vi "Do Request.vi"(7 "Processing In":refnum<class "Processing.lvclass">, 11 "Test HTTPS Controller in":refnum<class "Test HTTPS Controller.lvclass">) -> (0 "error out":errorcluster, 5 "Processing":refnum<class "Processing.lvclass">)   [LabVIEW 2020, in "Test HTTPS Controller.lvclass"]
uses:
  Test HTTPS Controller.lvclass
  HTTP Server/Processing/Processing.lvclass
  HTTP Server/Processing/Processing.lvclass/Processing.ctl
  <vilib>/IlluminatedG/IG HTTP Utils/HTTP Utils/Response/Response.lvclass
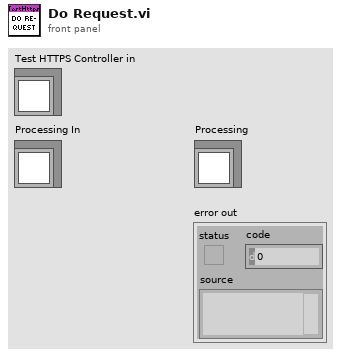
[diagram p1: front panel]
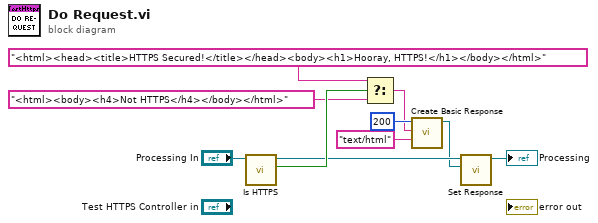
[diagram p0: block diagram]
diagram:
  n1 = call "Is HTTPS.vi"("Processing in"="Processing In") -> ("HTTPS?"=w9:bool, "Processing out"=w4:refnum<class "Processing.lvclass">)  [unwired: 8 in, 1 out]
  n2 = Select(t="<html><head><title>HTTPS Secured!</title></head><body><h1>Hooray, HTTPS!</h1></body></html>", s=w9, f="<html><body><h4>Not HTTPS</h4></body></html>") -> (s? t:f=w5:string)
  n3 = call <vilib>:"Create Basic Response.vi"("Content-Type (text/plain)"="text/html", "Payload"=w5, "Status Code"=u16 200) -> ("Response out"=w3:refnum<class "Response.lvclass">)  [unwired: 7 in, 1 out]
  n4 = call "Set Response.vi"("Response"=w3, "Processing in"=w4) -> ("Processing out"=→"Processing":refnum<class "Processing.lvclass">)  [unwired: 9 in]
